vi "PKDAQRunningAvg.vi"(9 "Block Data":T2, 10 "CountPoints":i32, 11 "CurPoints":i32) -> (1 "RunningAverages":T1)   [LabVIEW 2013]
uses:
  ctl/SummaryData.ctl
  ctl/BlockData.ctl
  <vilib>/Analysis/baseanly.llb/Mean (DBL).vi
  <vilib>/Analysis/NI_AALBase.lvlib
panel:
  in  "RunningAveragesIn":T1
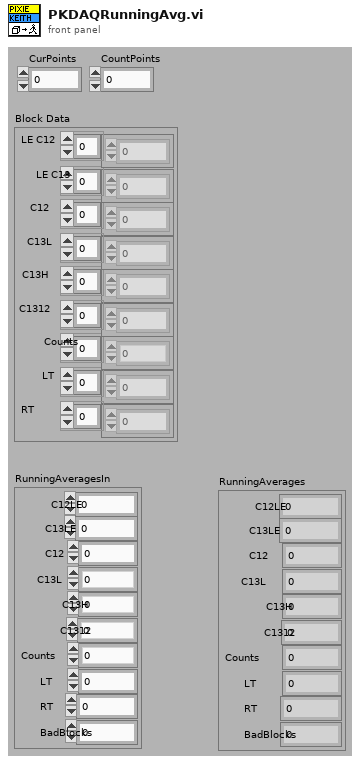
[diagram p1: front panel]
types:
  T1 = typedef "SummaryData.ctl" = cluster{"C12LE":dbl, "C13LE":dbl, "C12":dbl, "C13L":dbl, "C13H":dbl, "C1312":dbl, "Counts":u32, "LT":dbl, "RT":dbl, "BadBlocks":u8}
  T2 = typedef "BlockData.ctl" = cluster{"LE C12":dbl[], "LE C13":dbl[], "C12":dbl[], "C13L":dbl[], "C13H":dbl[], "C1312":dbl[], "Counts":u32[], "LT":dbl[], "RT":dbl[]}
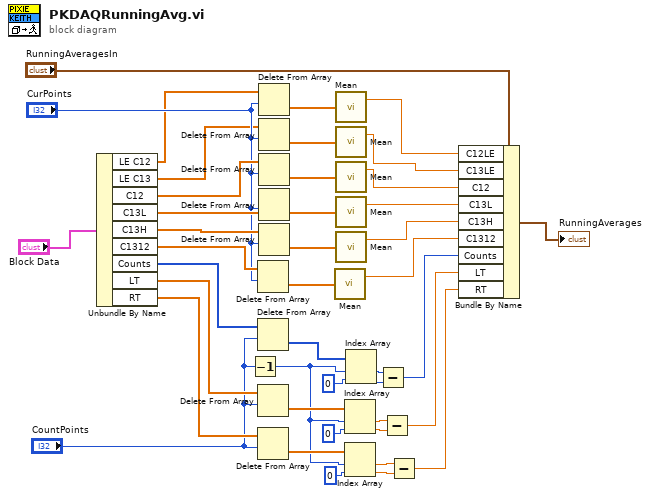
[diagram p0: block diagram]
diagram:
  n1 = Unbundle By Name("Block Data") -> ("LE C12"=w4:dbl[], "LE C13"=w3:dbl[], "C12"=w33:dbl[], "C13L"=w31:dbl[], "C13H"=w32:dbl[], "C1312"=w10:dbl[], "Counts"=w37:u32[], "LT"=w36:dbl[], "RT"=w35:dbl[])
  n2 = Decrement(x="CountPoints") -> (x-1=w12:i32)
  n3 = Delete From Array(array=w10, length="CurPoints") -> (deleted portion=w11:dbl[])  [unwired: 1 in, 1 out]
  n4 = Delete From Array(array=w37, length="CountPoints") -> (deleted portion=w27:u32[])  [unwired: 1 in, 1 out]
  n5 = Delete From Array(array=w36, length="CountPoints") -> (deleted portion=w16:dbl[])  [unwired: 1 in, 1 out]
  n6 = Delete From Array(array=w35, length="CountPoints") -> (deleted portion=w15:dbl[])  [unwired: 1 in, 1 out]
  n7 = Delete From Array(array=w4, length="CurPoints") -> (deleted portion=w7:dbl[])  [unwired: 1 in, 1 out]
  n8 = Delete From Array(array=w3, length="CurPoints") -> (deleted portion=w6:dbl[])  [unwired: 1 in, 1 out]
  n9 = Delete From Array(array=w33, length="CurPoints") -> (deleted portion=w30:dbl[])  [unwired: 1 in, 1 out]
  n10 = Delete From Array(array=w31, length="CurPoints") -> (deleted portion=w29:dbl[])  [unwired: 1 in, 1 out]
  n11 = Delete From Array(array=w32, length="CurPoints") -> (deleted portion=w28:dbl[])  [unwired: 1 in, 1 out]
  n12 = call-poly <vilib>:"Mean.vi"("X"=w11) -> ("mean"=w9:dbl)  [unwired: 1 out]
  n13 = call-poly <vilib>:"Mean.vi"("X"=w7) -> ("mean"=w2:dbl)  [unwired: 1 out]
  n14 = call-poly <vilib>:"Mean.vi"("X"=w6) -> ("mean"=w1:dbl)  [unwired: 1 out]
  n15 = call-poly <vilib>:"Mean.vi"("X"=w30) -> ("mean"=w40:dbl)  [unwired: 1 out]
  n16 = call-poly <vilib>:"Mean.vi"("X"=w29) -> ("mean"=w39:dbl)  [unwired: 1 out]
  n17 = call-poly <vilib>:"Mean.vi"("X"=w28) -> ("mean"=w38:dbl)  [unwired: 1 out]
  n18 = Index Array(array=w16, index #1=w12, index #2=0 ("index")) -> (element #1=w21:dbl, element #2=w22:dbl)
  n19 = Index Array(array=w15, index #1=w12, index #2=0 ("index")) -> (element #1=w18:dbl, element #2=w19:dbl)
  n20 = Index Array(array=w27, index #1=w12, index #2=0 ("index")) -> (element #1=w25:u32, element #2=w26:u32)
  n21 = Subtract(x=w25, y=w26) -> (x-y=w23:u32)
  n22 = Subtract(x=w21, y=w22) -> (x-y=w8:dbl)
  n23 = Subtract(x=w18, y=w19) -> (x-y=w13:dbl)
  n24 = Bundle By Name(cluster="RunningAveragesIn", "C12LE"=w2, "C13LE"=w1, "C12"=w40, "C13L"=w39, "C13H"=w38, "C1312"=w9, "Counts"=w23, "LT"=w8, "RT"=w13) -> (→"RunningAverages":T1)
